vi "Update Pullup Mode.vi"   [LabVIEW 2014, in "SLSC configuration Shared.lvlib"]
doc: "Updates the pull-up resitor mode on the pins."
uses:
  SLSC configuration Shared.lvlib
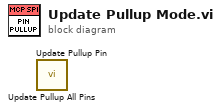
[diagram p0: block diagram]
diagram:
  n1 = call "Update Pullup All Pins.vi"() -> ()  [unwired: 9 in, 3 out]
  n2 = call "Update Pullup Pin.vi"() -> ()  [unwired: 9 in, 3 out]
